vi "Read nbrStepsInProfile.vi"(11 "TestMonitor in":refnum<class "TestMonitor.lvclass">) -> (2 "nbrStepsInProfile":u32 min=1, 3 "TestMonitor out":refnum<class "TestMonitor.lvclass">)   [LabVIEW 2015]
uses:
  TestMonitor.lvclass
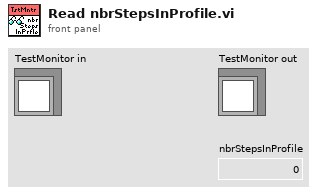
[diagram p1: front panel]
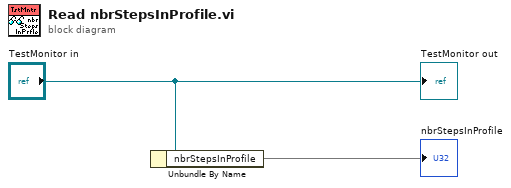
[diagram p0: block diagram]
diagram:
  n1 = Unbundle By Name("TestMonitor in") -> ("nbrStepsInProfile"=→"nbrStepsInProfile")
  "TestMonitor out" <- "TestMonitor in"
